vi "PersonnelJSONTest.vi"() -> (0 "error out":errorcluster, 2 "Pass":bool)   [LabVIEW 2015]
uses:
  Personnel/PersonnelType.ctl
  Personnel/Personnel.lvclass
panel:
  in  "Name":string
  in  "UniqueID":string
  in  "Role":T1
  in  "error in (no error)":errorcluster
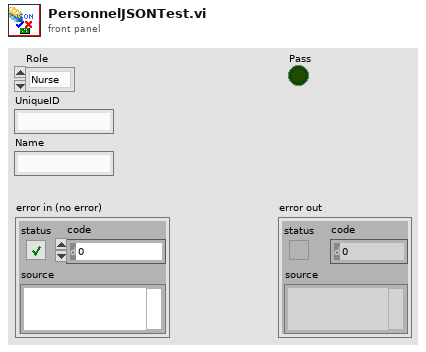
[diagram p1: front panel]
types:
  T1 = typedef "Personnel.lvclass/PersonnelType.ctl" = enum16{"Nurse", "Doctor", "Cleanning", "Admin"}
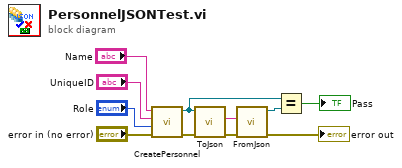
[diagram p0: block diagram]
diagram:
  n1 = call "CreatePersonnel.vi"("error in (no error)"="error in (no error)", "Role"="Role", "UniqueID"="UniqueID", "Name"="Name") -> ("error out"=w11:errorcluster, "output cluster"=w4:refnum<class "Personnel.lvclass">)  [unwired: 6 in]
  n2 = call "ToJson.vi"("error in (no error)"=w11, "Personnel in"=w4) -> ("error out"=w10:errorcluster, "PersonnelJson"=w9:string)  [unwired: 7 in, 1 out]
  n3 = call "FromJson.vi"("error in (no error)"=w10, "PersonnelJson"=w9) -> ("error out"=→"error out":errorcluster, "Personnel out"=w3:refnum<class "Personnel.lvclass">)  [unwired: 8 in]
  n4 = Equal?(x=w4, y=w3) -> (x = y?=→"Pass":bool)
